vi "Finish.vi"   [LabVIEW 2018]
doc: "This VI is called just before exiting. It is expected to close I/O refnum, save collected data, etc."
uses:
  <vilib>/Rock Robotics/WPI/Utilities/WPI_GetSetVariantRefNum.vi
types:
  T1 = typedef "WPI_CounterDevRef.ctl" = cluster{"DevStatus":errorcluster, "CntIndex":T2}
  T2 = typedef "FPGA_CounterCtrSystemIndex.ctl" = enum8{"Ctr 0", "Ctr 1", "Ctr 2", "Ctr 3", "Ctr 4", "Ctr 5", "Ctr 6", "Ctr 7", "Invalid"}
  T3 = typedef "WPI_SwitchDevRef.ctl" = cluster{"DevStatus":errorcluster, "DIO Channel":T4, "CntIndex":T2, "Normally Closed":bool}
  T4 = typedef "FPGA_DIOChannel.ctl" = enum8{"DIO 0", "DIO 1", "DIO 2", "DIO 3", "DIO 4", "DIO 5", "DIO 6", "DIO 7", "DIO 8", "DIO 9", "DIO MXP 0", "DIO MXP 1", "DIO MXP 2", "DIO MXP 3", "DIO MXP 4", "DIO MXP 5", "DIO MXP 6", "DIO MXP 7", "DIO MXP 8", "DIO MXP 9", "DIO MXP 10", "DIO MXP 11", "DIO MXP 12", "DIO MXP 13", "DIO MXP 14", "DIO MXP 15", "SPI Port CS1", "SPI Port CS2", "SPI Port CS3", "SPI Port MISO", "SPI Port MOSI", "Invalid"}
  T5 = typedef "WPI_JoystickDevRef.ctl" = cluster{"Device":T6}
  T6 = typedef "WPI_JoystickDeviceEnum.ctl" = enum16{"USB 0", "USB 1", "USB 2", "USB 3", "USB 4", "USB 5"}
  T7 = typedef "WPI_RobotDriveDevRef.ctl" = cluster{"DevStatus":errorcluster, "Motors[]":T8[], "Square Inputs":bool, "Max Output":dbl}
  T8 = typedef "WPI_MotorControlDeviceRef.ctl" = cluster{"DeviceStatus":errorcluster, "Type":T9, "PWM":cluster{"PWM Channel":T10, "DeadBand":T11}, "CAN":cluster{"Device Number":u8, "SetOutput VI Ref":variant, "GetOutput VI Ref":variant, "Enable VI Ref":variant, "Disable VI Ref":variant, "Data":variant}, "Invert":bool, "DIO PWM":cluster{"PWM \"Enable\" Channel":T10, "DIOChannel":T4, "PWM Rate":dbl}}
  T9 = typedef "WPI_MotorControlType.ctl" = enum16{"PWM", "CAN", "DIO PWM"}
  T10 = typedef "FPGA_DIOPWMChannel.ctl" = enum8{"PWM 0", "PWM 1", "PWM 2", "PWM 3", "PWM 4", "PWM 5", "PWM 6", "PWM 7", "PWM 8", "PWM 9", "PWM MXP 0", "PWM MXP 1", "PWM MXP 2", "PWM MXP 3", "PWM MXP 4", "PWM MXP 5", "PWM MXP 6", "PWM MXP 7", "PWM MXP 8", "PWM MXP 9", "Invalid"}
  T11 = typedef "WPI_PWMDeadband.ctl" = cluster{"Name":string, "maxPositivePwm":i32, "minPositivePwm":i32, "centerPwm":i32, "maxNegativePwm":i32, "minNegativePwm":i32, "angularRange":u16}
  T12 = typedef "WPI_SolenoidDevRef.ctl" = cluster{"DevStatus":errorcluster, "Pneumatics Control Module":u8, "Forward Solenoid Channel":T13, "Reverse Solenoid Channel":T13}
  T13 = typedef "WPI_SolenoidChannel.ctl" = enum8{"Solenoid 0", "Solenoid 1", "Solenoid 2", "Solenoid 3", "Solenoid 4", "Solenoid 5", "Solenoid 6", "Solenoid 7", "Invalid"}
  T14 = typedef "WPI_EncoderDevRef.ctl" = cluster{"DevStatus":errorcluster, "EncoderIndex":T15, "CounterIndex":T2, "DistancePerCount":dbl, "Decoding Type":T16}
  T15 = typedef "FPGA_EncoderIdx.ctl" = enum8{"Enc 0", "Enc 1", "Enc 2", "Enc 3", "Enc 4", "Enc 5", "Enc 6", "Enc 7", "Invalid"}
  T16 = typedef "WPI_EncoderType.ctl" = enum16{"1x", "2x", "4x"}
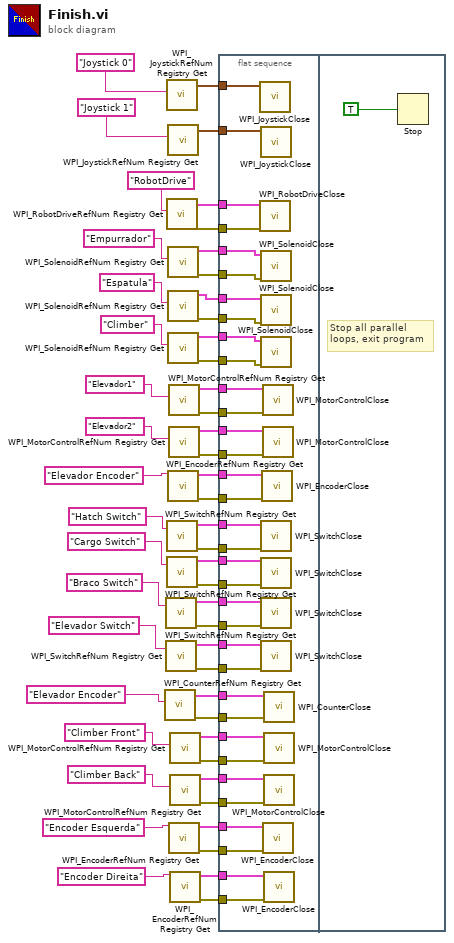
[diagram p0: block diagram]
diagram:
  n1 = call <vilib>:"WPI_CounterRefNum Registry Get.vi"("refnum name"="Elevador Encoder") -> ("error out"=w14:errorcluster, "CounterDevRef"=w15:T1)  [unwired: 9 in]
  n2 = call <vilib>:"WPI_SwitchRefNum Registry Get.vi"("refnum name"="Braco Switch") -> ("error out"=w20:errorcluster, "SwitchDevRef"=w21:T3)  [unwired: 9 in]
  n3 = call <vilib>:"WPI_SwitchRefNum Registry Get.vi"("refnum name"="Elevador Switch") -> ("error out"=w18:errorcluster, "SwitchDevRef"=w19:T3)  [unwired: 9 in]
  n4 = call <vilib>:"WPI_JoystickRefNum Registry Get.vi"("refnum name"="Joystick 0") -> ("JoystickDevRef"=w44:T5)  [unwired: 1 in, 9 out]
  n5 = call <vilib>:"WPI_RobotDriveRefNum Registry Get.vi"("refnum name"="RobotDrive") -> ("error out"=w41:errorcluster, "RobotDriveDevRef"=w42:T7)  [unwired: 1 in, 8 out]
  n6 = call <vilib>:"WPI_SwitchRefNum Registry Get.vi"("refnum name"="Hatch Switch") -> ("error out"=w22:errorcluster, "SwitchDevRef"=w23:T3)  [unwired: 9 in]
  n7 = call <vilib>:"WPI_SwitchRefNum Registry Get.vi"("refnum name"="Cargo Switch") -> ("error out"=w16:errorcluster, "SwitchDevRef"=w17:T3)  [unwired: 9 in]
  n8 = call <vilib>:"WPI_JoystickRefNum Registry Get.vi"("refnum name"="Joystick 1") -> ("JoystickDevRef"=w43:T5)  [unwired: 1 in, 9 out]
  n9 = call <vilib>:"WPI_SolenoidRefNum Registry Get.vi"("refnum name"="Empurrador") -> ("error out"=w39:errorcluster, "SolenoidDevRef"=w40:T12)  [unwired: 9 in]
  n10 = call <vilib>:"WPI_SolenoidRefNum Registry Get.vi"("refnum name"="Espatula") -> ("error out"=w37:errorcluster, "SolenoidDevRef"=w38:T12)  [unwired: 9 in]
  n11 = call <vilib>:"WPI_SolenoidRefNum Registry Get.vi"("refnum name"="Climber") -> ("error out"=w35:errorcluster, "SolenoidDevRef"=w36:T12)  [unwired: 9 in]
  n12 = call <vilib>:"WPI_EncoderRefNum Registry Get.vi"("refnum name"="Elevador Encoder") -> ("error out"=w28:errorcluster, "EncoderDevRef"=w29:T14)  [unwired: 9 in]
  n13 = call <vilib>:"WPI_MotorControlRefNum Registry Get.vi"("refnum name"="Elevador1") -> ("error out"=w33:errorcluster, "MotorControlDevRef"=w34:T8)  [unwired: 9 in]
  n14 = call <vilib>:"WPI_MotorControlRefNum Registry Get.vi"("refnum name"="Elevador2") -> ("error out"=w31:errorcluster, "MotorControlDevRef"=w32:T8)  [unwired: 9 in]
  n15 = call <vilib>:"WPI_EncoderRefNum Registry Get.vi"("refnum name"="Encoder Esquerda") -> ("error out"=w6:errorcluster, "EncoderDevRef"=w5:T14)  [unwired: 9 in]
  n16 = call <vilib>:"WPI_MotorControlRefNum Registry Get.vi"("refnum name"="Climber Front") -> ("error out"=w10:errorcluster, "MotorControlDevRef"=w9:T8)  [unwired: 9 in]
  n17 = call <vilib>:"WPI_MotorControlRefNum Registry Get.vi"("refnum name"="Climber Back") -> ("error out"=w12:errorcluster, "MotorControlDevRef"=w11:T8)  [unwired: 9 in]
  n18 = call <vilib>:"WPI_EncoderRefNum Registry Get.vi"("refnum name"="Encoder Direita") -> ("error out"=w1:errorcluster, "EncoderDevRef"=w2:T14)  [unwired: 9 in]
  n19 = flat-sequence {
    tunnel: w44 -> [w86]
    tunnel: w43 -> [w85]
    tunnel: w42 -> [w84]
    tunnel: w41 -> [w83]
    tunnel: w40 -> [w82]
    tunnel: w39 -> [w81]
    tunnel: w38 -> [w80]
    tunnel: w37 -> [w79]
    tunnel: w36 -> [w78]
    tunnel: w35 -> [w77]
    tunnel: w34 -> [w76]
    tunnel: w33 -> [w75]
    tunnel: w32 -> [w74]
    tunnel: w31 -> [w73]
    tunnel: w29 -> [w72]
    tunnel: w28 -> [w71]
    tunnel: w23 -> [w70]
    tunnel: w22 -> [w69]
    tunnel: w21 -> [w68]
    tunnel: w20 -> [w67]
    tunnel: w19 -> [w66]
    tunnel: w18 -> [w65]
    tunnel: w17 -> [w64]
    tunnel: w16 -> [w63]
    tunnel: w15 -> [w62]
    tunnel: w14 -> [w61]
    tunnel: w9 -> [w57]
    tunnel: w10 -> [w58]
    tunnel: w11 -> [w59]
    tunnel: w12 -> [w60]
    tunnel: w5 -> [w55]
    tunnel: w6 -> [w56]
    tunnel: w2 -> [w54]
    tunnel: w1 -> [w53]
    frame #0 {
      n20 = call <vilib>:"WPI_JoystickClose.vi"("JoystickDevRef"=w86) -> ()  [unwired: 11 out]
      n21 = call <vilib>:"WPI_RobotDriveClose.vi"("error in (no error)"=w83, "RobotDriveDevRef"=w84) -> ()  [unwired: 10 out]
      n22 = call <vilib>:"WPI_JoystickClose.vi"("JoystickDevRef"=w85) -> ()  [unwired: 11 out]
      n23 = call <vilib>:"WPI_SolenoidClose.vi"("error in (no error)"=w81, "SolenoidDevRef"=w82) -> ()  [unwired: 9 in, 1 out]
      n24 = call <vilib>:"WPI_SolenoidClose.vi"("error in (no error)"=w79, "SolenoidDevRef"=w80) -> ()  [unwired: 9 in, 1 out]
      n25 = call <vilib>:"WPI_SolenoidClose.vi"("error in (no error)"=w77, "SolenoidDevRef"=w78) -> ()  [unwired: 9 in, 1 out]
      n26 = call <vilib>:"WPI_SwitchClose.vi"("error in (no error)"=w69, "SwitchDevRef"=w70) -> ()  [unwired: 9 in, 1 out]
      n27 = call <vilib>:"WPI_SwitchClose.vi"("error in (no error)"=w63, "SwitchDevRef"=w64) -> ()  [unwired: 9 in, 1 out]
      n28 = call <vilib>:"WPI_SwitchClose.vi"("error in (no error)"=w67, "SwitchDevRef"=w68) -> ()  [unwired: 9 in, 1 out]
      n29 = call <vilib>:"WPI_SwitchClose.vi"("error in (no error)"=w65, "SwitchDevRef"=w66) -> ()  [unwired: 9 in, 1 out]
      n30 = call <vilib>:"WPI_EncoderClose.vi"("error in (no error)"=w71, "EncoderDevRef"=w72) -> ()  [unwired: 9 in, 1 out]
      n31 = call <vilib>:"WPI_MotorControlClose.vi"("error in"=w75, "MotorControlDevRef"=w76) -> ()  [unwired: 9 in, 1 out]
      n32 = call <vilib>:"WPI_MotorControlClose.vi"("error in"=w73, "MotorControlDevRef"=w74) -> ()  [unwired: 9 in, 1 out]
      n33 = call <vilib>:"WPI_EncoderClose.vi"("error in (no error)"=w56, "EncoderDevRef"=w55) -> ()  [unwired: 9 in, 1 out]
      n34 = call <vilib>:"WPI_CounterClose.vi"("error in (no error)"=w61, "CounterDevRef"=w62) -> ()  [unwired: 9 in, 1 out]
      n35 = call <vilib>:"WPI_MotorControlClose.vi"("error in"=w58, "MotorControlDevRef"=w57) -> ()  [unwired: 9 in, 1 out]
      n36 = call <vilib>:"WPI_MotorControlClose.vi"("error in"=w60, "MotorControlDevRef"=w59) -> ()  [unwired: 9 in, 1 out]
      n37 = call <vilib>:"WPI_EncoderClose.vi"("error in (no error)"=w53, "EncoderDevRef"=w54) -> ()  [unwired: 9 in, 1 out]
    }
    frame #1 {
      # "Stop all parallel\nloops, exit program"
      n38 = Stop(stop? (T)=TRUE ("Quit")) -> ()
    }
  }
